vi "RTD Temperature Monitor.vi"() -> ()   [LabVIEW 2010]
panel:
  out "Reading":bool
  out "Waiting":bool
  in  "Measurement Target":T1(ring)
  out "Temp (C)":dbl
  out "RTD Ohms":dbl
  in  "Take Reading":bool
  in  "Time between Readings (S)":dbl=2.0
  in  "Continuous Read":bool=TRUE
  in  "Exit":bool
  # "AlgoStim ETS Temperature Monitor"
  # "This tool makes use of the same RTD\nresistance measurement techniques,\nfixture measurement switch paths\nand software conversion functions as\nare used in the Board Level and Final\nFunctional Electrical Tests to deter-\nmine reference temperatures."
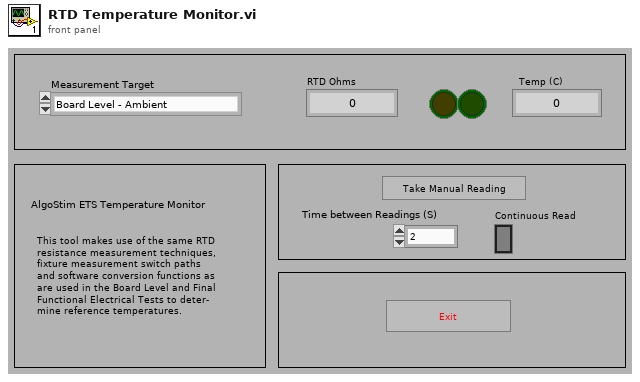
[diagram p1: front panel]
types:
  T1 = enum16{"Board Level - Ambient", "Board Level - Cavity 1", "Device Level - Ambient", "Device Level - Test Block", "Device Level - Cavity 1", "Device Level - Cavity 2"}
  T2 = typedef "niSE SessionRefnum.ctl" = refnum<k1>
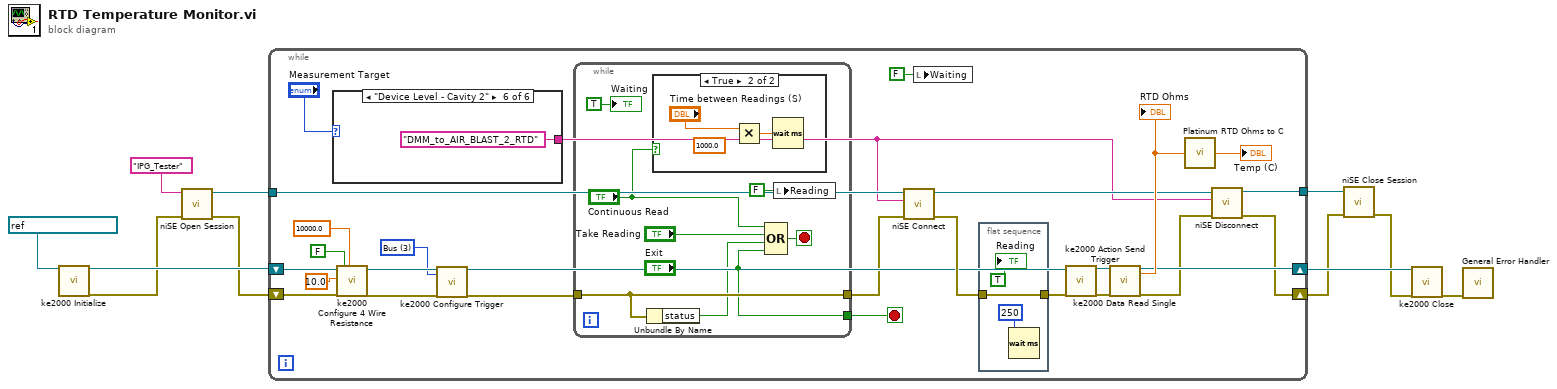
[diagram p0: block diagram]
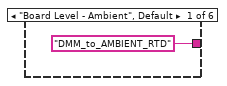
[diagram p2: hidden frame]
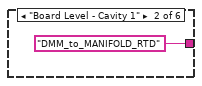
[diagram p3: hidden frame]
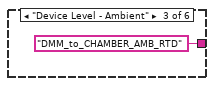
[diagram p4: hidden frame]
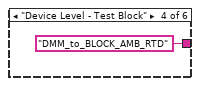
[diagram p5: hidden frame]
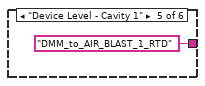
[diagram p6: hidden frame]
diagram:
  n1 = call "ke2000 Initialize.vi"("VISA resource name"=refnum<visa-resource-name> "GPIB0::8::INSTR") -> ("VISA resource name out"=w8:refnum<visa-resource-name>, "error out"=w6:errorcluster)  [unwired: 17 in]
  n2 = call <vilib>:"niSE Open Session.vi"("error in (no error)"=w6, "Virtual Device Name (SwitchConfiguration1)"="IPG_Tester") -> ("error out"=w5:errorcluster, "NISE Session (out)"=w4:T2)  [unwired: 4 in]
  n3 = while {
    shift-right: [w34] -> w10
    shift-left: w8 -> [w22]
    shift-right: [w16] -> w3
    shift-left: w5 -> [w23]
    tunnel: w4 -> [w17]
    tunnel: [w15] -> w1
    stop <- w31 stop-if-true
    w26 = u16 3 items=["Immediate", "Timer", "Manual", "Bus", "External"] ("Source (0: Immediate)")
    n4 = case shown="\"Device Level - Cavity 2\"" "Measurement Target" {
      tunnel: ["DMM_to_AMBIENT_RTD" ("Connection Specification (\"\")") "DMM_to_MANIFOLD_RTD" ("Connection Specification (\"\")") "DMM_to_CHAMBER_AMB_RTD" ("Connection Specification (\"\")") "DMM_to_BLOCK_AMB_RTD" ("Connection Specification (\"\")") "DMM_to_AIR_BLAST_1_RTD" ("Connection Specification (\"\")") "DMM_to_AIR_BLAST_2_RTD" ("Connection Specification (\"\")")] -> w13
      frame "Board Level - Ambient", Default {
      }
      frame "Board Level - Cavity 1" {
      }
      frame "Device Level - Ambient" {
      }
      frame "Device Level - Test Block" {
      }
      frame "Device Level - Cavity 1" {
      }
      frame "Device Level - Cavity 2" {
      }
    }
    n5 = call "ke2000 Configure 4 Wire Resistance.vi"("VISA resource name"=w22, "Power Line Cycles (1.00)"=10.0, "error in (no error)"=w23, "Auto Range? (T: Auto)"=FALSE, "Custom Range (0 Ohm)"=10000.0) -> ("VISA resource name out"=w28:refnum<visa-resource-name>, "error out"=w27:errorcluster)  [unwired: 13 in]
    n6 = call "ke2000 Configure Trigger.vi"("VISA resource name"=w28, "Source (0: Immediate)"=w26, "error in (no error)"=w27) -> ("VISA resource name out"=w21:refnum<visa-resource-name>, "error out"=w20:errorcluster)  [unwired: 15 in]
    n7 = while {
      tunnel: w20 -> [w52]
      tunnel: [w52] -> w18
      tunnel: ["Exit"] -> w31
      stop <- w55 stop-if-true
      n8 = Unbundle By Name(w52) -> ("status"=w50:bool)
      n9 = case shown="True" "Continuous Read" {
        frame False {
        }
        frame True {
          n10 = Multiply(x="Time between Readings (S)", y=1000.0) -> (x*y=w58:dbl)
          n11 = Wait (ms)(milliseconds to wait=w58) -> ()  [unwired: 1 out]
        }
      }
      n12 = Compound Arithmetic op=OR("Continuous Read", "Take Reading", w50, "Exit") -> (w55:bool)
      n13 = local write "Reading"(FALSE ("Reading")) -> ()
      "Waiting" <- TRUE ("Waiting")
    }
    n14 = call <vilib>:"niSE Connect.vi"("error in (no error)"=w18, "Connection Specification (\"\")"=w13, "NISE Session (in)"=w17) -> ("error out"=w29:errorcluster, "NISE Session (out)"=w32:T2)  [unwired: 7 in]
    n15 = local write "Waiting"(FALSE ("Waiting")) -> ()
    n16 = flat-sequence {
      tunnel: [w46] -> w30
      tunnel: w29 -> [w46]
      frame #0 {
        n17 = Wait (ms)(milliseconds to wait=u32 250) -> ()  [unwired: 1 out]
        "Reading" <- TRUE ("Reading")
      }
    }
    n18 = call "ke2000 Action Send Trigger.vi"("VISA resource name"=w21, "error in (no error)"=w30) -> ("VISA resource name out"=w37:refnum<visa-resource-name>, "error out"=w38:errorcluster)  [unwired: 16 in]
    n19 = call "ke2000 Data Read Single.vi"("VISA resource name"=w37, "error in (no error)"=w38) -> ("VISA resource name out"=w34:refnum<visa-resource-name>, "Measurement"=w36:dbl, "error out"=w33:errorcluster)  [unwired: 13 in, 2 out]
    "RTD Ohms" <- w36
    n20 = call "Platinum RTD Ohms to C.vi"("Rt"=w36) -> ("Temp (C)"=→"Temp (C)":dbl)
    n21 = call <vilib>:"niSE Disconnect.vi"("error in (no error)"=w33, "Disconnection Specification (\"\")"=w13, "NISE Session (in)"=w32) -> ("error out"=w16:errorcluster, "NISE Session (out)"=w15:T2)  [unwired: 3 in]
  }
  n22 = call <vilib>:"niSE Close Session.vi"("error in (no error)"=w3, "NISE Session (in)"=w1) -> ("error out"=w2:errorcluster)  [unwired: 5 in]
  n23 = call "ke2000 Close.vi"("VISA resource name"=w10, "error in (no error)"=w2) -> ("error out"=w9:errorcluster)  [unwired: 17 in]
  n24 = call <vilib>:"General Error Handler.vi"("error in (no error)"=w9) -> ()  [unwired: 10 in, 5 out]
